vi "Write Test Info.vi"(8 "error in (no error)":errorcluster, 10 "Test Info":refnum<vi>, 11 "Auto UI in":refnum<class "Auto UI.lvclass">) -> (0 "error out":errorcluster, 3 "Auto UI out":refnum<class "Auto UI.lvclass">)   [LabVIEW 2023, in "GUI.lvlib" / "Auto UI.lvlib" / "Auto UI.lvclass"]
uses:
  Auto UI.lvclass
  Typdefs/Auto GUI/Test Info.ctl
  Auto UI.lvclass/Auto UI.ctl
  GUI.lvlib
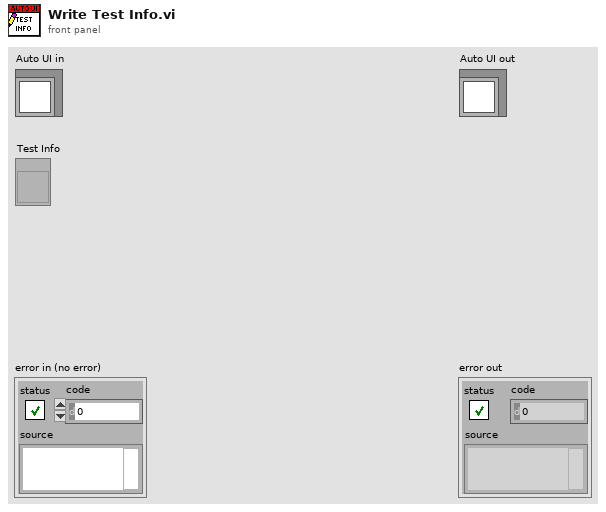
[diagram p1: front panel]
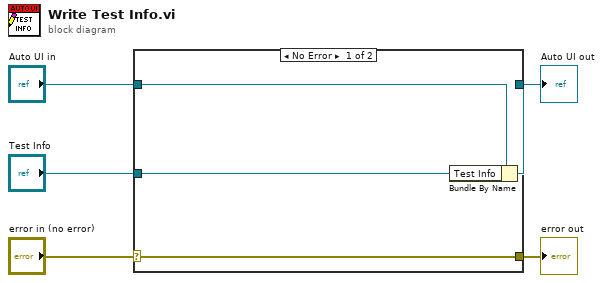
[diagram p0: block diagram]
diagram:
  n1 = case shown="No Error" "error in (no error)" {
    selector: "error in (no error)" -> [w9 w10]
    tunnel: [w9 w10] -> w4
    tunnel: [w7 w11] -> w2
    tunnel: "Auto UI in" -> [w8 w11]
    tunnel: "Test Info" -> [w6 _]
    frame No Error {
      n2 = Bundle By Name(cluster=w8, "Test Info"=w6) -> (w7:refnum<class "Auto UI.lvclass">)
    }
    frame Error {
    }
  }
  "error out" <- w4
  "Auto UI out" <- w2
